vi "START.vi"(11 "hDevice输入":i32) -> (3 "hDevice":i32)   [LabVIEW 2012]
uses:
  PCI8521_32.dll
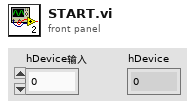
[diagram p1: front panel]
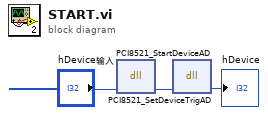
[diagram p0: block diagram]
diagram:
  n1 = dll-call lib="PCI8521_32.dll" fn="PCI8521_StartDeviceAD" label="StartDeviceAD"("hDevice"="hDevice输入") -> ("hDevice"=w2:i32)  [unwired: 4 in, 2 out]
  n2 = dll-call lib="PCI8521_32.dll" fn="PCI8521_SetDeviceTrigAD" ("SetDeviceTrigAD")("hDevice"=w2) -> ("hDevice"=→"hDevice":i32)  [unwired: 4 in, 2 out]
